vi "Configure Trace Operation (Exchange,Copy).vi"(0 "VISA resource name":refnum<visa-resource-name>, 5 "Trace 1 (1: Trace 1)":u16(ring)=1 items=["Trace 1"=1, "Trace 2"=2, "Trace 3"=3], 7 "Operation (2: Exchange)":u16(ring)=2 items=["Exchange"=2, "Copy"=3], 9 "Trace 2 (2: Trace 2)":u16(ring)=2 items=["Trace 1"=1, "Trace 2"=2, "Trace 3"=3, "Display Line"=4], 11 "error in (no error)":errorcluster) -> (4 "VISA resource name out":refnum<visa-resource-name>, 15 "error out":errorcluster)   [LabVIEW 2014, in "Agilent ESA PSA Series.lvlib"]
doc: "Configures the type of trace to acquire."
uses:
  Agilent ESA PSA Series.lvlib
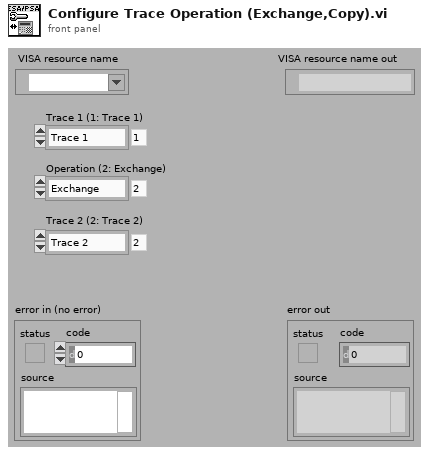
[diagram p1: front panel]
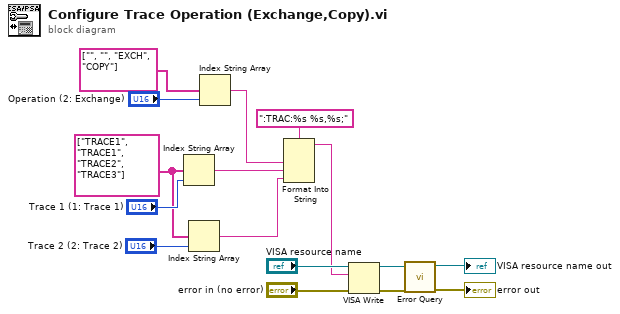
[diagram p0: block diagram]
diagram:
  w8 = string[] ["TRACE1", "TRACE1", "TRACE2", "TRACE3"]
  n1 = Index String Array(1:"Trace 1 (1: Trace 1)", 2:w8) -> (0:w3:string)  [unwired: 1 in]
  n2 = Index String Array(1:"Trace 2 (2: Trace 2)", 2:w8) -> (0:w2:string)  [unwired: 1 in]
  n3 = Index String Array(1:"Operation (2: Exchange)", 2:string[] ["", "", "EXCH", "COPY"]) -> (0:w5:string)  [unwired: 1 in]
  n4 = Format Into String(format string=":TRAC:%s %s,%s;", w5, w3, w2) -> (resulting string=w1:string)  [unwired: 2 in, 1 out]
  n5 = VISA Write(VISA resource name="VISA resource name", write buffer=w1, error in (no error)="error in (no error)") -> (VISA resource name out=w14:refnum<visa-resource-name>, error out=w12:errorcluster)  [unwired: 1 out]
  n6 = call "Error Query.vi"("error in (no error)"=w12, "VISA resource name"=w14) -> ("error out"=→"error out":errorcluster, "VISA resource name out"=→"VISA resource name out":refnum<visa-resource-name>)  [unwired: 6 in, 2 out]
